vi "SDSU_cmdAddMngr.vi"(9 "cmds in":T1[](array[typedef]), 10 "action":enum16{"find", "get", "set"}(ring)=enum."get", 11 "argument":string) -> (1 "cmd":T1, 2 "cmdadds":T1[](array[typedef]), 3 "found":bool)   [LabVIEW 2016]
uses:
  SDSU_cmdTableEntry.ctl
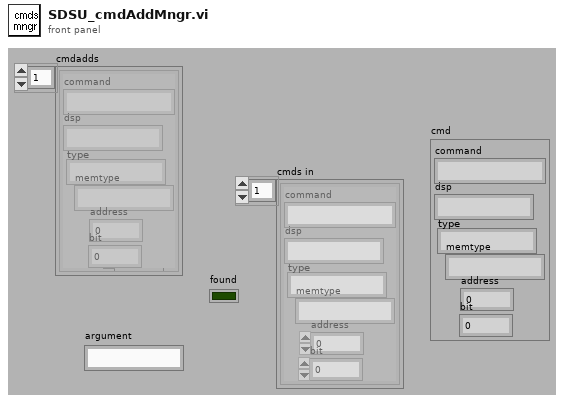
[diagram p1: front panel]
types:
  T1 = typedef "SDSU_cmdTableEntry.ctl" = cluster{"command":string, "dsp":string, "type":string, "memtype":string, "address":i32, "bit":i32}
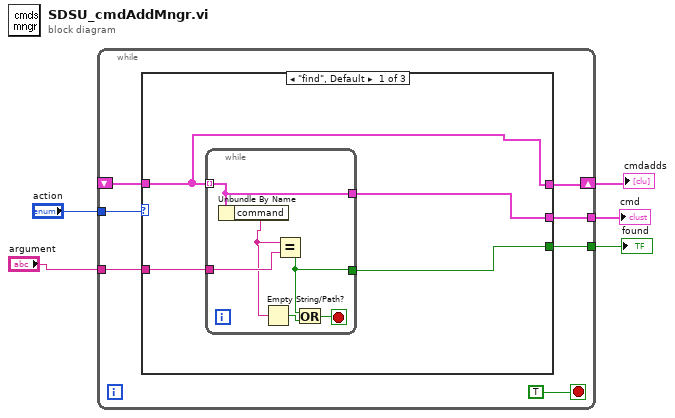
[diagram p0: block diagram]
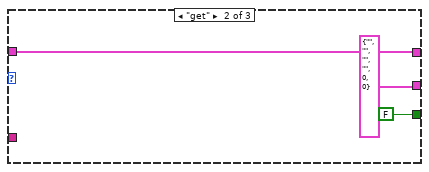
[diagram p2: hidden frame]
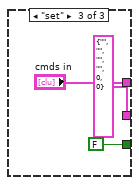
[diagram p3: hidden frame]
diagram:
  n1 = while {
    tunnel: "action" -> [w11]
    shift-right: [w10] -> w4
    shift-left: _ -> [w9]
    tunnel: "argument" -> [w8]
    tunnel: [w7] -> w2
    tunnel: [w6] -> w1
    stop <- TRUE stop-if-true
    n2 = case shown="\"find\", Default" w11 {
      tunnel: [w13 w25 "cmds in"] -> w10
      tunnel: w9 -> [w13 w25 _]
      tunnel: w8 -> [w16 _ _]
      tunnel: [w15 FALSE FALSE] -> w7
      tunnel: [w14 T1 {"command"="", "dsp"="", "type"="", "memtype"="", "address"=0, "bit"=0} ("Cluster") T1 {"command"="", "dsp"="", "type"="", "memtype"="", "address"=0, "bit"=0} ("Cluster")] -> w6
      frame "find", Default {
        n3 = while {
          tunnel: w13 -> [w18] mode=indexing
          tunnel: w16 -> [w22]
          tunnel: [w19] -> w15
          tunnel: [w18] -> w14
          stop <- w21 stop-if-true
          n4 = Unbundle By Name(w18) -> ("command"=w20:string)
          n5 = Empty String/Path?(string/path=w20) -> (empty?=w17:bool)
          n6 = Equal?(x=w20, y=w22) -> (x = y?=w19:bool)
          n7 = Or(x=w19, y=w17) -> (x .or. y?=w21:bool)
        }
      }
      frame "get" {
      }
      frame "set" {
      }
    }
  }
  "cmdadds" <- w4
  "found" <- w2
  "cmd" <- w1
